vi "Format (Internal).vi"(7 "call chain format params":T1, 8 "error in (no error)":errorcluster, 10 "log record":T2 {"timestamp" format="%<%x %.3X>T"}, 11 "format string":string) -> (0 "error out":errorcluster, 3 "formatted string":string)   [LabVIEW 2024, in "Logging.lvlib" / "Format String.lvclass"]
uses:
  Format String.lvclass
  Log Record.ctl
  Logger/Internal Log Levels.ctl
  Call Chain Format Parameters.ctl
  Logging.lvlib
panel:
  # "Connector Pane"
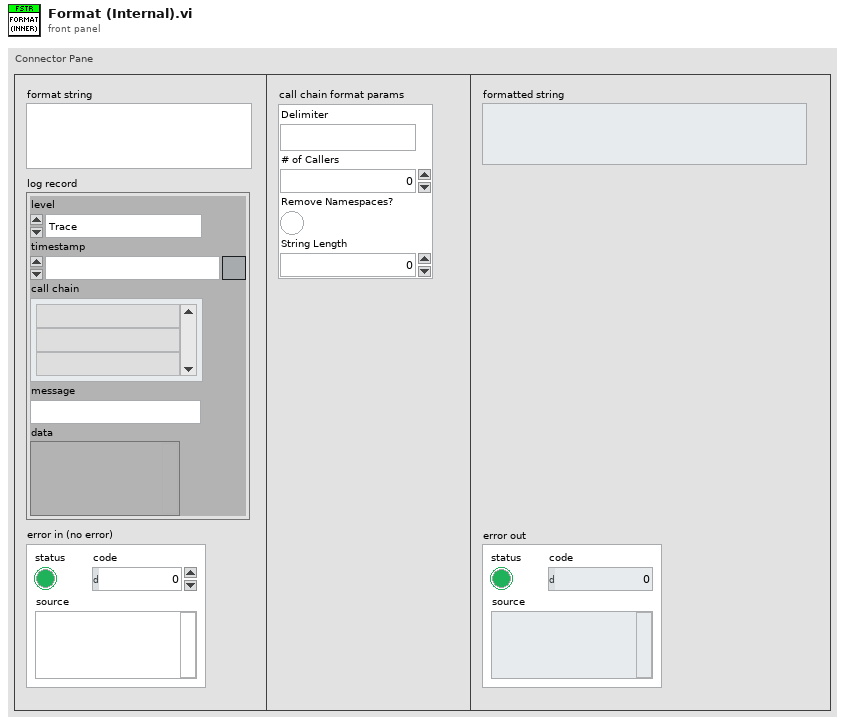
[diagram p1: front panel]
types:
  T1 = typedef "Logging.lvlib/Format String.lvclass/Call Chain Format Parameters.ctl" = cluster{"Delimiter":string, "# of Callers":i32, "Remove Namespaces?":bool, "String Length":i32}
  T2 = typedef "Logging.lvlib/Log Record.ctl" = cluster{"level":T3, "timestamp":timestamp, "call chain":string[], "message":string, "data":variant}
  T3 = typedef "Logging.lvlib/Internal Log Levels.ctl" = enum16{"Trace", "Debug", "Info", "Warning", "Error", "Critical", "Internal"}
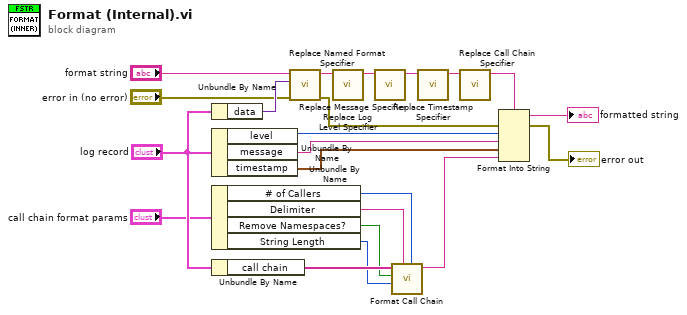
[diagram p0: block diagram]
diagram:
  n1 = Unbundle By Name("log record") -> ("data"=w3:variant)
  n2 = Unbundle By Name("log record") -> ("level"=w19:T3, "message"=w20:string, "timestamp"=w16:timestamp)
  n3 = Unbundle By Name("call chain format params") -> ("# of Callers"=w8:i32, "Delimiter"=w9:string, "Remove Namespaces?"=w7:bool, "String Length"=w6:i32)
  n4 = Unbundle By Name("log record") -> ("call chain"=w12:string[])
  n5 = call "Replace Named Format Specifier.vi"("error in (no error)"="error in (no error)", "data"=w3, "format string"="format string") -> ("error out"=w2:errorcluster, "resulting string"=w4:string)  [unwired: 7 in]
  n6 = call "Replace Log Level Specifier.vi"("format string"=w4) -> ("resulting string"=w18:string)  [unwired: 10 in]
  n7 = call "Replace Message Specifier.vi"("format string"=w18) -> ("resulting string"=w15:string)  [unwired: 10 in]
  n8 = call "Format Call Chain.vi"("number of callers (-1: all)"=w8, "delimiter (\" > \")"=w9, "string length (-1: none)"=w6, "remove namespaces? (T)"=w7, "call chain"=w12) -> ("formatted call chain"=w11:string)  [unwired: 6 in]
  n9 = call "Replace Timestamp Specifier.vi"("format string"=w15) -> ("resulting string"=w14:string)  [unwired: 10 in]
  n10 = call "Replace Call Chain Specifier.vi"("format string"=w14) -> ("resulting string"=w13:string)  [unwired: 10 in]
  n11 = Format Into String(format string=w13, error in=w2, w19, w20, w16, w11) -> (resulting string=→"formatted string":string, error out=→"error out":errorcluster)  [unwired: 1 in]
